vi "加载application.vi"(8 "error in (no error)":errorcluster caption="错误输入（无错误）") -> (0 "error out":errorcluster caption="错误输出")   [LabVIEW 2014]
doc: "加载应用信息"
uses:
  R/manifest.vi
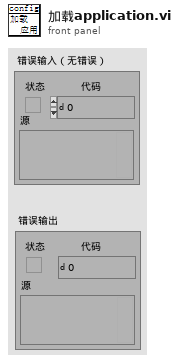
[diagram p1: front panel]
types:
  T1 = cluster{"应用状态":bool, "vi名称":string, "刷新间隔":u32, "显示数据精度":u32, "储存数据精度":u32}
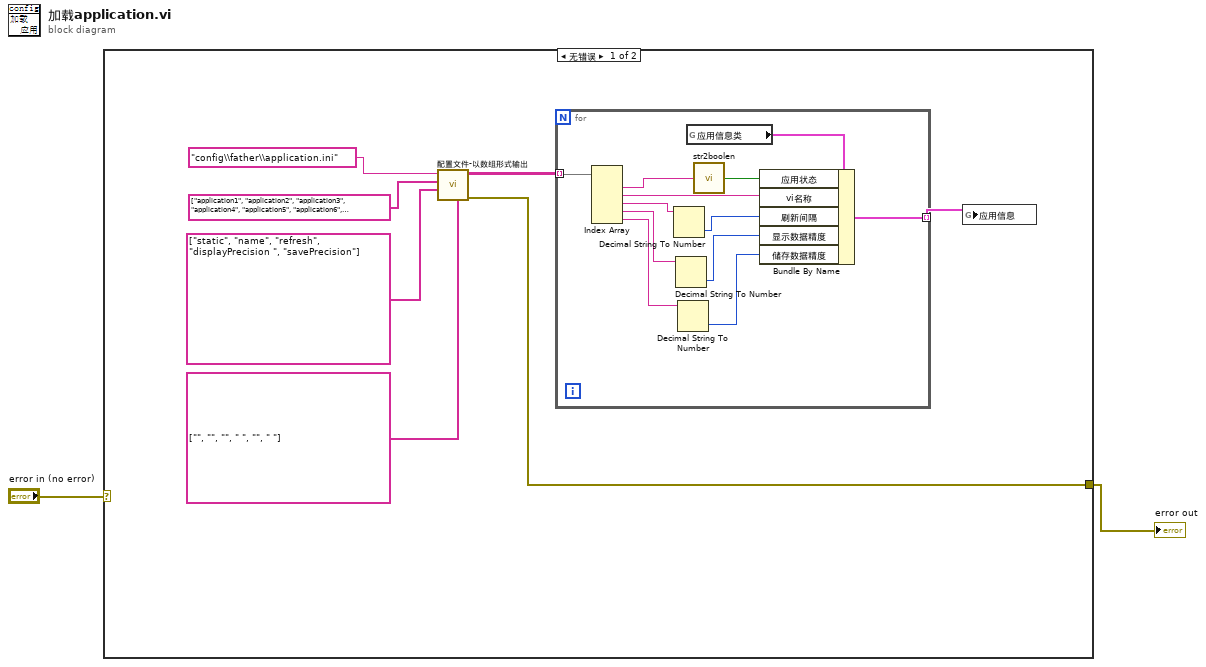
[diagram p0: block diagram]
diagram:
  n1 = case shown="无错误" "error in (no error)" {
    selector: "error in (no error)" -> [_ w22]
    tunnel: [w3 w22] -> w1
    frame No Error {
      n2 = call "配置文件-以数组形式输出.vi"("默认值"=string[] ["", "", "", " ", "", " "] ("键名"), "键名"=string[] ["static", "name", "refresh", "displayPrecision ", "savePrecision"], "章名"=string[] ["application1", "application2", "application3", "application4", "application5", "application6", "application7", "application8"], "路径"="config\\father\\application.ini") -> ("error out"=w3:errorcluster, "输出值"=w5:string[][])  [unwired: 6 in]
      n3 = for {
        tunnel: w5 -> [w21] mode=indexing
        tunnel: [w10] -> w4 mode=indexing
        n4 = Index Array(array=w21) -> (element #1=w19:string, element #2=w17:string, element #3=w16:string, element #4=w14:string, element #5=w12:string)  [unwired: 5 in]
        n5 = Decimal String To Number(string=w16) -> (number=w15:i32)  [unwired: 2 in, 1 out]
        n6 = Decimal String To Number(string=w14) -> (number=w13:i32)  [unwired: 2 in, 1 out]
        n7 = Decimal String To Number(string=w12) -> (number=w11:i32)  [unwired: 2 in, 1 out]
        n8 = global read "类信息.vi" "应用信息类"() -> (w20:T1)
        n9 = call "str2boolen.vi"("Str"=w19) -> ("Boolen"=w18:bool)
        n10 = Bundle By Name(cluster=w20, "应用状态"=w18, "vi名称"=w17, "刷新间隔"=w15, "显示数据精度"=w13, "储存数据精度"=w11) -> (w10:T1)
      }
      n11 = global write "manifest.vi" "应用信息"(w4) -> ()
    }
    frame Error {
    }
  }
  "error out" <- w1
